vi "Flatten Readable.vi"(11 "Lockin SR830.lvclass":refnum<class "Lockin SR830.lvclass">) -> ()   [LabVIEW 2023, in "Lockin SR830.lvclass"]
uses:
  Lockin SR830.lvclass
  Control Panel.vi
  Global/File Locations.vi
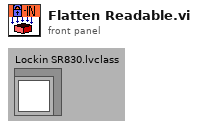
[diagram p1: front panel]
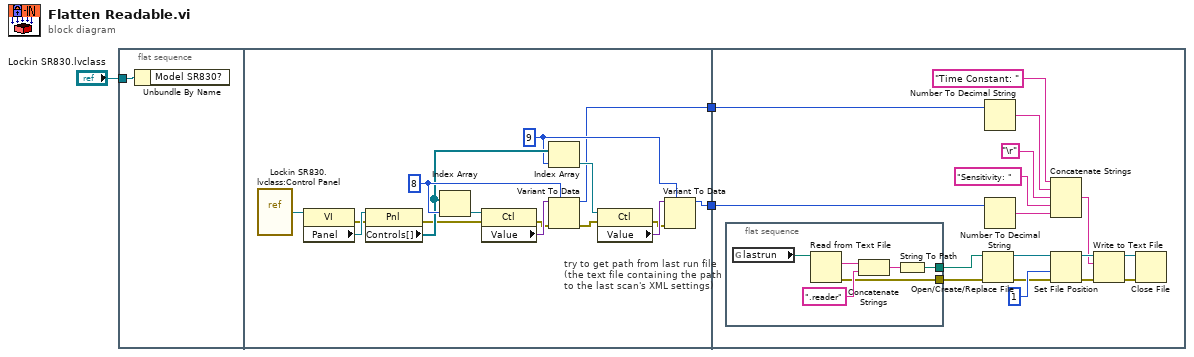
[diagram p0: block diagram]
diagram:
  n1 = flat-sequence {
    tunnel: "Lockin SR830.lvclass" -> [w4]
    tunnel: [w10] -> w2
    tunnel: [w9] -> w1
    tunnel: w2 -> [w25]
    tunnel: w1 -> [w21]
    frame #0 {
      n2 = Unbundle By Name(w4) -> ()  [unwired: 1 out]
    }
    frame #1 {
      w11 = 9
      w16 = 8
      n3 = vi-ref "Lockin SR830.lvclass:Control Panel.vi"() -> (w20:refnum<vi>)
      n4 = property class="VI"(reference=w20) -> (error out=w18:errorcluster, "Panel"=w19:refnum<vi>)  [unwired: 1 in, 1 out]
      n5 = property class="Pnl"(reference=w19, error in=w18) -> (error out=w8:errorcluster, "Controls[]"=w14:refnum<vi>[])  [unwired: 1 out]
      n6 = Index Array(array=w14, index=w16) -> (element=w17:refnum<vi>)
      n7 = property class="Ctl"(reference=w17, error in=w8) -> (error out=w7:errorcluster, "Value"=w15:variant)  [unwired: 1 out]
      n8 = Index Array(array=w14, index=w11) -> (element=w13:refnum<vi>)
      n9 = Variant To Data(error in=w7, type=w16, Variant=w15) -> (data=w10:i32, error out=w6:errorcluster)
      n10 = property class="Ctl"(reference=w13, error in=w6) -> (error out=w5:errorcluster, "Value"=w12:variant)  [unwired: 1 out]
      n11 = Variant To Data(error in=w5, type=w11, Variant=w12) -> (data=w9:i32)  [unwired: 1 out]
    }
    frame #2 {
      n12 = flat-sequence "try to get path from last run file\n(the text file containing the path\nto the last scan's XML settings)" {
        tunnel: [w43] -> w32
        tunnel: [w38] -> w37
        frame #0 {
          n13 = global read "File Locations.vi" "lastrun"() -> (w42:path)
          n14 = Read from Text File(file (use dialog)=w42) -> (text=w41:string, error out=w38:errorcluster)  [unwired: 1 in, 4 out]
          n15 = Concatenate Strings(w41, ".reader") -> (w39:string)
          n16 = String To Path(string=w39) -> (path=w43:path)
        }
      }
      n17 = Open/Create/Replace File(file path (use dialog)=w32, error in=w37) -> (refnum out=w36:refnum<file>, error out=w34:errorcluster)  [unwired: 4 in, 1 out]
      n18 = Number To Decimal String(number=w25) -> (decimal integer string=w24:string)  [unwired: 1 in]
      n19 = Number To Decimal String(number=w21) -> (decimal integer string=w22:string)  [unwired: 1 in]
      n20 = Concatenate Strings("Time Constant: ", w24, "\r", "Sensitivity: ", w22) -> (w28:string)
      n21 = Set File Position(refnum=w36, from (0:start)=1, error in=w34) -> (refnum out=w31:refnum<file>, error out=w33:errorcluster)  [unwired: 1 in]
      n22 = Write to Text File(file (use dialog)=w31, text=w28, error in=w33) -> (refnum out=w30:refnum<file>, error out=w29:errorcluster)  [unwired: 1 in, 1 out]
      n23 = Close File(refnum=w30, error in=w29) -> ()  [unwired: 2 out]
    }
  }
